vi "Do Write.vi"(8 "error in (no error)":errorcluster, 10 "Interface":refnum<class "Interface.lvclass">, 11 "Section 2 in":refnum<class "Section 2.lvclass">) -> (0 "error out":errorcluster, 3 "Section 2 out":refnum<class "Section 2.lvclass">, 4 "All Keys Found?":bool)   [LabVIEW 2014, in "LVOOP Introduction.lvlib" / "Section 2.lvclass"]
doc: "Write keys/value pairs to Interface.\n\nOverwriting dynamic dispatch VI."
uses:
  Section 2.lvclass
  Configuration/Classes/Interface/Interface.lvclass
  Section 2.lvclass/Section 2.ctl
  Configuration/Classes/Section/Section.lvclass
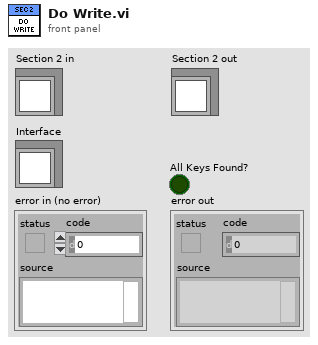
[diagram p1: front panel]
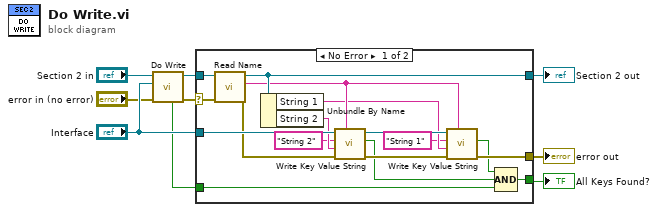
[diagram p0: block diagram]
diagram:
  n1 = call-parent "Do Write.vi"("error in (no error)"="error in (no error)", "Interface"="Interface", "Section in"="Section 2 in") -> ("error out"=w3:errorcluster, "Section out"=w4:refnum<class "Section 2.lvclass">, "All Keys Found?"=w1:bool)  [unwired: 6 in]
  n2 = case shown="No Error" w3 {
    selector: w3 -> [w11 w27]
    tunnel: w4 -> [w12 w28]
    tunnel: [w26 w28] -> w9
    tunnel: "Interface" -> [w25 _]
    tunnel: [w18 w27] -> w8
    tunnel: [w13 _] -> w7
    tunnel: w1 -> [w10 _]
    frame No Error {
      n3 = call "Read Name.vi"("error in (no error)"=w11, "Section in"=w12) -> ("error out"=w22:errorcluster, "Name"=w19:string, "Section out"=w26:refnum<class "Section 2.lvclass">)  [unwired: 7 in]
      n4 = Unbundle By Name(w26) -> ("String 1"=w15:string, "String 2"=w24:string)
      n5 = call-dynamic "Write Key Value String.vi"("Section Name"=w19, "error in (no error)"=w22, "Value"=w24, "Key Name"="String 2", "Interface in"=w25) -> ("error out"=w20:errorcluster, "found"=w16:bool, "Interface out"=w21:refnum<class "Interface.lvclass">)  [unwired: 4 in]
      n6 = call-dynamic "Write Key Value String.vi"("Section Name"=w19, "error in (no error)"=w20, "Value"=w15, "Key Name"="String 1", "Interface in"=w21) -> ("error out"=w18:errorcluster, "found"=w17:bool)  [unwired: 4 in, 1 out]
      n7 = Compound Arithmetic op=AND(w17, w16, w10) -> (w13:bool)
    }
    frame Error {
    }
  }
  "error out" <- w8
  "Section 2 out" <- w9
  "All Keys Found?" <- w7
